vi "Registry.vi"(6 "Registry Configuration":T2, 7 "Command (Get)":T4, 8 "Use Regex? (F)":bool, 9 "UniqueName Object (Set)":refnum<class "UniqueName.lvclass">, 10 "Search term (Get & Delete Operations)":string, 11 "Key (FQN)":T3) -> (0 "Found or Completed?":bool, 1 "Returned Object":refnum<class "UniqueName.lvclass">, 2 "Multiple Match?":bool, 3 "Returned Objects":refnum<class "UniqueName.lvclass">[](array[class]), 4 "Registry Status":T1)   [LabVIEW 2014, in "UniqueName.lvlib" / "UniqueName.lvclass"]
uses:
  UniqueName.lvclass
  Command.ctl
  Key.ctl
  RegistryConfiguration.ctl
  Delimiter/Delimiter.lvclass
  RandomStringGenerator/RandomStringGenerator.lvclass
  UniquenessCriteria/UniquenessCriteria.lvclass
  NameIncrementAlgorithm/StringIncrementAlgorithm.lvclass
  RegistryStatus.ctl
  UniqueName.lvclass/UniqueName.ctl
  <vilib>/regexp/Match Regular Expression.xnode
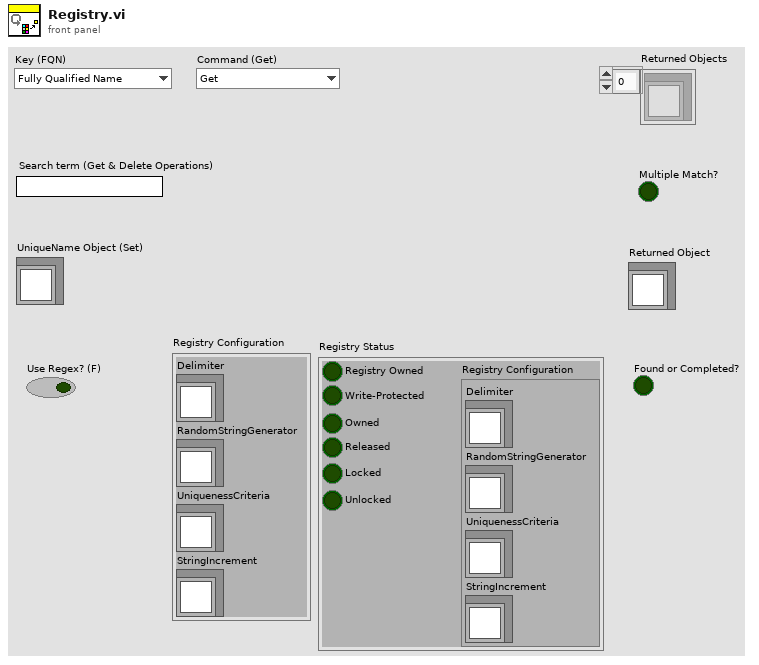
[diagram p1: front panel]
types:
  T1 = typedef "UniqueName.lvlib/UniqueName.lvclass/RegistryStatus.ctl" = cluster{"Registry Configuration":T2, "Registry Owned":bool, "Write-Protected":bool, "Owned":bool, "Released":bool, "Locked":bool, "Unlocked":bool}
  T2 = typedef "UniqueName.lvlib/UniqueName.lvclass/RegistryConfiguration.ctl" = cluster{"Delimiter":refnum<class "Delimiter.lvclass">, "RandomStringGenerator":refnum<class "RandomStringGenerator.lvclass">, "UniquenessCriteria":refnum<class "UniquenessCriteria.lvclass">, "StringIncrement":refnum<class "StringIncrementAlgorithm.lvclass">}
  T3 = typedef "UniqueName.lvlib/UniqueName.lvclass/Key.ctl" = enum16{"Fully Qualified Name", "Unique Name", "Given Name", "Parent Fully Qualified Name"}
  T4 = typedef "UniqueName.lvlib/UniqueName.lvclass/Command.ctl" = enum16{"Get", "Get All", "Set", "Delete", "Get Status", "Init", "Reserve Ownership", "Release Ownership", "Lock", "Unlock"}
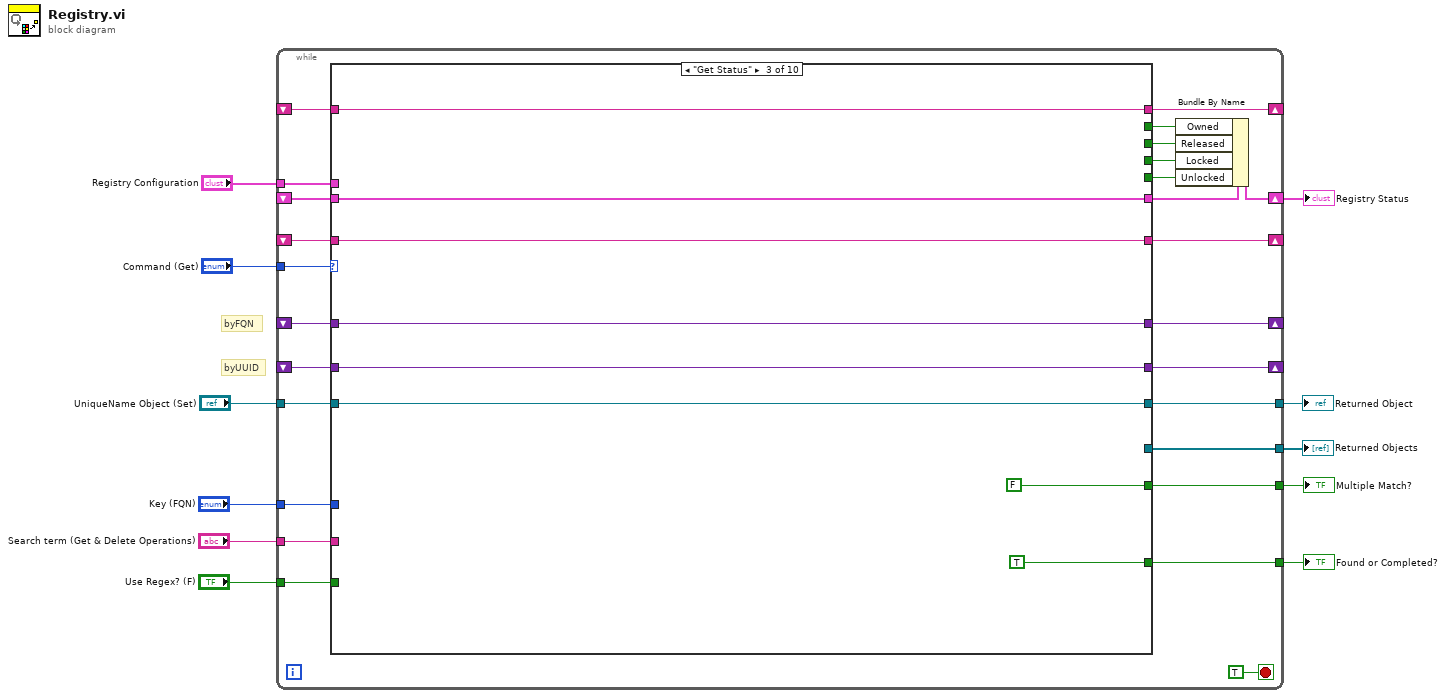
[diagram p0: block diagram]
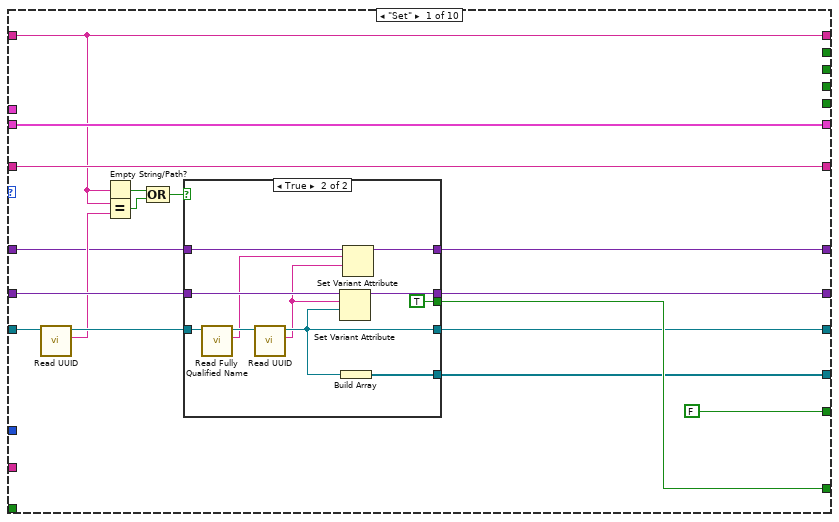
[diagram p2: hidden frame]
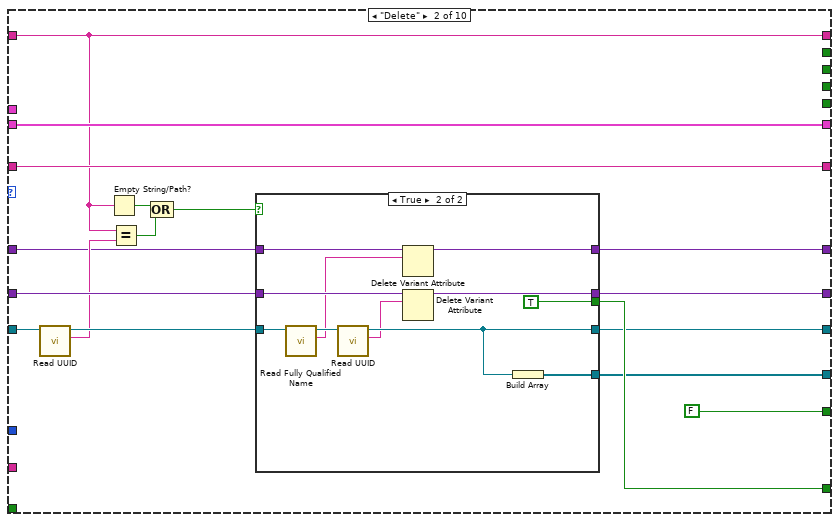
[diagram p4: hidden frame]
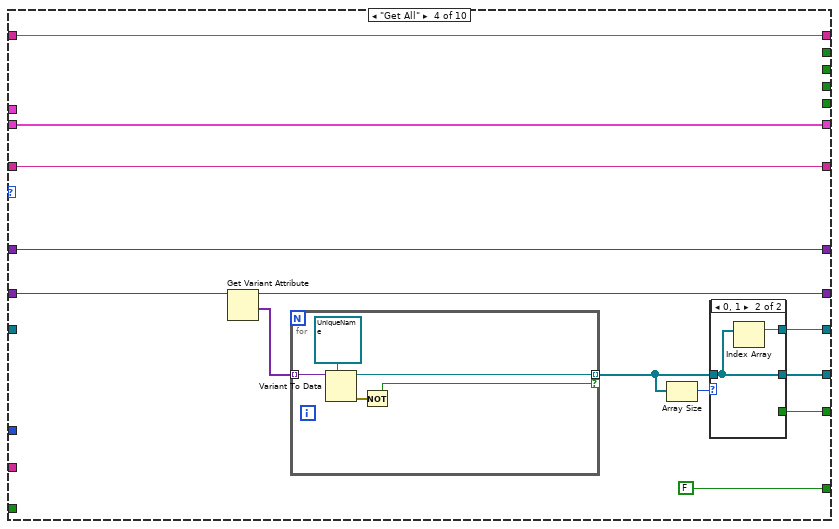
[diagram p6: hidden frame]
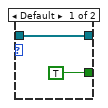
[diagram p7: hidden frame]
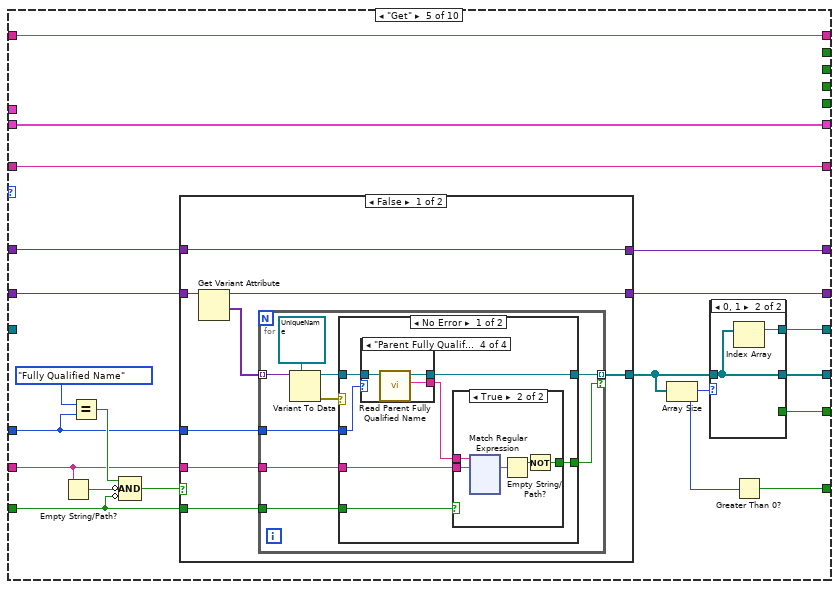
[diagram p8: hidden frame]
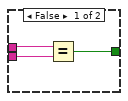
[diagram p9: hidden frame]
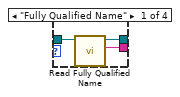
[diagram p10: hidden frame]
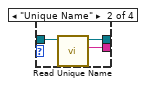
[diagram p11: hidden frame]
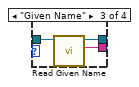
[diagram p12: hidden frame]
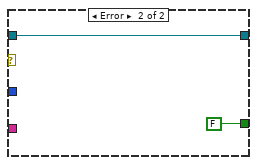
[diagram p13: hidden frame]
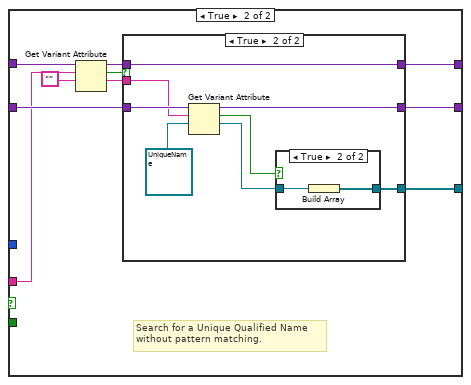
[diagram p14: hidden frame]
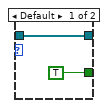
[diagram p17: hidden frame]
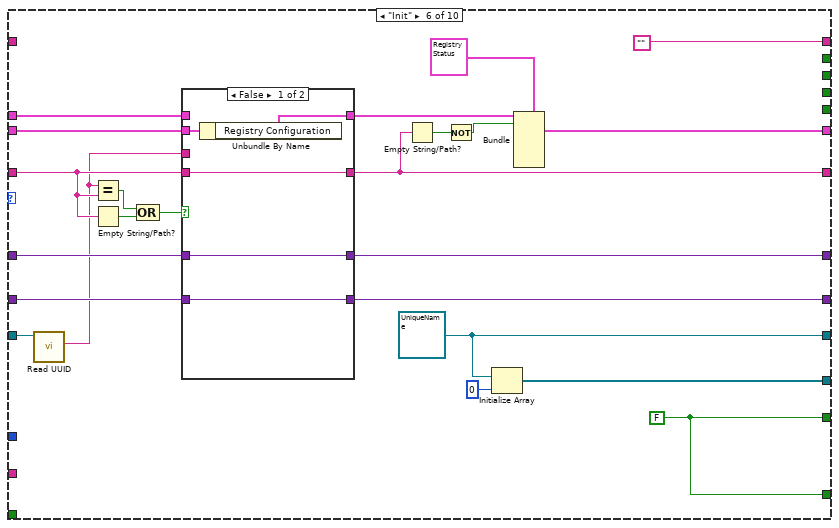
[diagram p18: hidden frame]
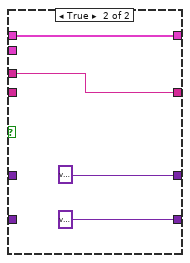
[diagram p19: hidden frame]
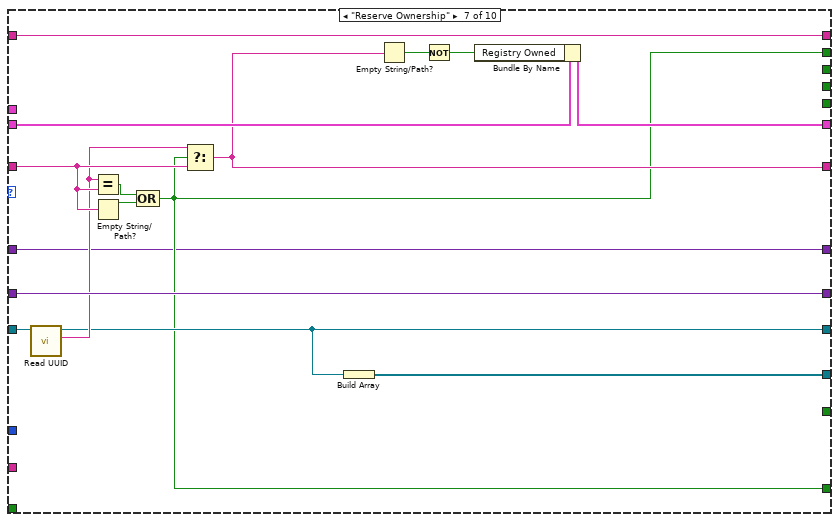
[diagram p20: hidden frame]
diagram:
  # "byUUID"
  # "byFQN"
  n1 = while {
    shift-right: [w35] -> _
    shift-left: _ -> [w33]
    tunnel: "Command (Get)" -> [w36]
    tunnel: "UniqueName Object (Set)" -> [w34]
    tunnel: [w32] -> w10
    tunnel: [w31] -> w9
    tunnel: [w30] -> w8
    tunnel: "Key (FQN)" -> [w29]
    tunnel: "Search term (Get & Delete Operations)" -> [w28]
    tunnel: [w27] -> w5
    tunnel: "Use Regex? (F)" -> [w26]
    shift-right: [w24] -> _
    shift-left: _ -> [w25]
    shift-right: [w19] -> w2
    shift-left: _ -> [w23]
    tunnel: "Registry Configuration" -> [w22]
    shift-right: [w20] -> _
    shift-left: _ -> [w21]
    shift-right: [w12] -> _
    shift-left: _ -> [w13]
    stop <- TRUE stop-if-true
    n2 = case shown="\"Get Status\"" w36 {
      tunnel: [w53 w83 w104 w116 w146 w356 w379 w396 w413 w429] -> w35
      tunnel: w34 -> [w46 w72 w105 _ _ w335 w371 w386 w401 w420]
      tunnel: w33 -> [w54 w84 w104 w117 w147 w348 w379 w396 w413 w429]
      tunnel: [w49 w80 w105 w110 w142 w355 w369 w385 w400 w415] -> w32
      tunnel: [w50 w77 _ w112 w144 w353 w368 _ _ w416] -> w31
      tunnel: [FALSE FALSE FALSE w111 w143 w352 _ _ _ FALSE] -> w30
      tunnel: w29 -> [_ _ _ _ w137 _ _ _ _ _]
      tunnel: w28 -> [_ _ _ _ w138 _ _ _ _ _]
      tunnel: [w52 w81 TRUE ("found") FALSE ("found") w134 w352 w367 w383 w398 w418] -> w27
      tunnel: w26 -> [_ _ _ _ w136 _ _ _ _ _]
      tunnel: w25 -> [w48 w79 w103 w109 w133 w347 w378 w395 w403 w428]
      tunnel: [w48 w79 w103 w109 w133 w341 w374 w395 w403 w423] -> w24
      tunnel: w23 -> [w47 w78 w102 w108 w132 w346 w376 w388 w405 w422]
      tunnel: [w47 w78 w102 w108 w132 w344 w375 w387 w404 w421] -> w18
      tunnel: w22 -> [_ _ _ _ _ w345 _ _ _ _]
      tunnel: w21 -> [w41 w75 w100 w107 w130 _ w377 w392 w410 w424]
      tunnel: [w41 w75 w100 w107 w130 "" w377 w389 w406 w424] -> w20
      tunnel: [_ _ _ _ _ _ _ w383 _ _] -> w17
      tunnel: [_ _ _ _ _ _ _ _ w398 _] -> w16
      tunnel: [_ _ _ _ _ _ w367 _ _ _] -> w15
      tunnel: [_ _ _ _ _ _ _ _ _ w418] -> w14
      tunnel: w13 -> [w39 w69 w99 w106 w129 w336 w366 w382 w397 w414]
      tunnel: [w38 w68 w99 w106 w128 w337 w366 w382 w397 w414] -> w12
      frame "Set" {
        n3 = call "Read UUID.vi"("UniqueName in"=w46) -> ("UUID"=w40:string, "UniqueName out"=w45:refnum<class "UniqueName.lvclass">)  [unwired: 9 in]
        n4 = Empty String/Path?(string/path=w41) -> (empty?=w42:bool)
        n5 = Equal?(x=w41, y=w40) -> (x = y?=w44:bool)
        n6 = Compound Arithmetic op=OR(w42, w44) -> (w43:bool)
        n7 = case shown="True" w43 {
          tunnel: w54 -> [w56 w67]
          tunnel: [w56 w66] -> w53
          tunnel: [_ TRUE ("replaced")] -> w52
          tunnel: w45 -> [_ w62]
          tunnel: [_ w65] -> w50
          tunnel: [_ w60] -> w49
          tunnel: w39 -> [w55 w63]
          tunnel: [w55 w57] -> w38
          frame False {
          }
          frame True {
            n8 = call "Read Fully Qualified Name.vi"("UniqueName in"=w62) -> ("Fully Qualified Name"=w59:string, "UniqueName out"=w61:refnum<class "UniqueName.lvclass">)  [unwired: 9 in]
            n9 = call "Read UUID.vi"("UniqueName in"=w61) -> ("UUID"=w58:string, "UniqueName out"=w60:refnum<class "UniqueName.lvclass">)  [unwired: 9 in]
            n10 = Set Variant Attribute(Variant=w67, name=w58, value=w60) -> (Variant out=w66:variant)  [unwired: 1 in, 2 out]
            n11 = Build Array(w60) -> (w65:refnum<class "UniqueName.lvclass">[])
            n12 = Set Variant Attribute(Variant=w63, name=w59, value=w58) -> (Variant out=w57:variant)  [unwired: 1 in, 2 out]
          }
        }
      }
      frame "Delete" {
        n13 = call "Read UUID.vi"("UniqueName in"=w72) -> ("UUID"=w70:string, "UniqueName out"=w71:refnum<class "UniqueName.lvclass">)  [unwired: 9 in]
        n14 = Empty String/Path?(string/path=w75) -> (empty?=w76:bool)
        n15 = Equal?(x=w75, y=w70) -> (x = y?=w74:bool)
        n16 = Compound Arithmetic op=OR(w76, w74) -> (w73:bool)
        n17 = case shown="True" w73 {
          tunnel: w71 -> [_ w90]
          tunnel: w84 -> [w86 w97]
          tunnel: [w86 w96] -> w83
          tunnel: [_ TRUE] -> w81
          tunnel: [_ w89] -> w80
          tunnel: [_ w94] -> w77
          tunnel: w69 -> [w85 w93]
          tunnel: [w85 w92] -> w68
          frame False {
          }
          frame True {
            n18 = call "Read Fully Qualified Name.vi"("UniqueName in"=w90) -> ("Fully Qualified Name"=w88:string, "UniqueName out"=w91:refnum<class "UniqueName.lvclass">)  [unwired: 9 in]
            n19 = call "Read UUID.vi"("UniqueName in"=w91) -> ("UUID"=w87:string, "UniqueName out"=w89:refnum<class "UniqueName.lvclass">)  [unwired: 9 in]
            n20 = Delete Variant Attribute(6:w88, 7:w93) -> (3:w92:variant)  [unwired: 1 in, 2 out]
            n21 = Delete Variant Attribute(6:w87, 7:w97) -> (3:w96:variant)  [unwired: 1 in, 2 out]
            n22 = Build Array(w89) -> (w94:refnum<class "UniqueName.lvclass">[])
          }
        }
      }
      frame "Get Status" {
      }
      frame "Get All" {
        n23 = Get Variant Attribute(Variant=w117) -> (duplicate Variant=w116:variant, values=w115:variant[])  [unwired: 3 in, 2 out]
        n24 = for {
          tunnel: w115 -> [w127] mode=indexing
          tunnel: [w125] -> w113 mode=indexing if=w123
          n25 = Variant To Data(type=refnum<class "UniqueName.lvclass"> refnum ("UniqueName.lvclass"), Variant=w127) -> (data=w125:refnum<class "UniqueName.lvclass">, error out=w124:errorcluster)  [unwired: 1 in]
          n26 = Not(x=w124) -> (.not. x?=w123:bool)
        }
        n27 = Array Size(array=w113) -> (size(s)=w114:i32)
        n28 = case shown="0, 1" w114 {
          tunnel: w113 -> [w120 w122]
          tunnel: [w120 w122] -> w112
          tunnel: [TRUE _] -> w111
          tunnel: [_ w121] -> w110
          frame Default {
          }
          frame 0, 1 {
            n29 = Index Array(array=w122) -> (element=w121:refnum<class "UniqueName.lvclass">)  [unwired: 1 in]
          }
        }
      }
      frame "Get" {
        n30 = Empty String/Path?(string/path=w138) -> (empty?=w141:bool)
        n31 = Equal?(x=Key."Fully Qualified Name", y=w137) -> (x = y?=w140:bool)
        n32 = Compound Arithmetic op=AND(w140, invert w141, invert w136) -> (w139:bool)
        n33 = case shown="False" w139 {
          tunnel: w147 -> [w155 w317]
          tunnel: [w154 w316] -> w146
          tunnel: [w153 w315] -> w145
          tunnel: w138 -> [w150 w312]
          tunnel: w137 -> [w149 _]
          tunnel: w136 -> [w151 _]
          tunnel: w129 -> [w148 w314]
          tunnel: [w148 w309] -> w128
          frame False {
            n34 = Get Variant Attribute(Variant=w155) -> (duplicate Variant=w154:variant, values=w152:variant[])  [unwired: 3 in, 2 out]
            n35 = for {
              tunnel: w152 -> [w164] mode=indexing
              tunnel: [w160] -> w153 mode=indexing if=w158
              tunnel: w151 -> [w157]
              tunnel: w150 -> [w156]
              tunnel: w149 -> [w162]
              n36 = Variant To Data(type=refnum<class "UniqueName.lvclass"> refnum ("UniqueName.lvclass"), Variant=w164) -> (data=w161:refnum<class "UniqueName.lvclass">, error out=w159:errorcluster)  [unwired: 1 in]
              n37 = case shown="No Error" w159 {
                tunnel: [w165 FALSE] -> w158
                tunnel: w162 -> [w171 _]
                tunnel: w161 -> [w170 w307]
                tunnel: [w169 w307] -> w160
                tunnel: w157 -> [w168 _]
                tunnel: w156 -> [w166 _]
                frame No Error {
                  n38 = case shown="\"Parent Fully Qualified Name\"" w171 {
                    tunnel: w170 -> [w296 w299 w302 w305]
                    tunnel: [w295 w298 w301 w304] -> w169
                    tunnel: [w294 w297 w300 w303] -> w167
                    frame "Fully Qualified Name" {
                      n39 = call "Read Fully Qualified Name.vi"("UniqueName in"=w296) -> ("Fully Qualified Name"=w294:string, "UniqueName out"=w295:refnum<class "UniqueName.lvclass">)  [unwired: 9 in]
                    }
                    frame "Unique Name" {
                      n40 = call "Read Unique Name.vi"("UniqueName in"=w299) -> ("Unique Name"=w297:string, "UniqueName out"=w298:refnum<class "UniqueName.lvclass">)  [unwired: 9 in]
                    }
                    frame "Given Name" {
                      n41 = call "Read Given Name.vi"("UniqueName in"=w302) -> ("Given Name"=w300:string, "UniqueName out"=w301:refnum<class "UniqueName.lvclass">)  [unwired: 9 in]
                    }
                    frame "Parent Fully Qualified Name" {
                      n42 = call "Read Parent Fully Qualified Name.vi"("UniqueName in"=w305) -> ("Parent Fully Qualified Name"=w303:string, "UniqueName out"=w304:refnum<class "UniqueName.lvclass">)  [unwired: 9 in]
                    }
                  }
                  n43 = case shown="True" w168 {
                    tunnel: w167 -> [w174 w179]
                    tunnel: w166 -> [w173 w178]
                    tunnel: [w172 w175] -> w165
                    frame False {
                      n44 = Equal?(x=w174, y=w173) -> (x = y?=w172:bool)
                    }
                    frame True {
                      n45 = xnode "Match Regular Expression"("input string"=w179, "regular expression"=w178) -> ("whole match"=w177:string)  [unwired: 4 in, 4 out]
                      n46 = Empty String/Path?(string/path=w177) -> (empty?=w176:bool)
                      n47 = Not(x=w176) -> (.not. x?=w175:bool)
                    }
                  }
                }
                frame Error {
                }
              }
            }
          }
          frame True {
            # "Search for a Unique Qualified Name\nwithout pattern matching."
            n48 = Get Variant Attribute(Variant=w314, name=w312, default value (empty Variant)="") -> (duplicate Variant=w308:variant, found=w310:bool, value=w311:string)  [unwired: 1 in, 1 out]
            n49 = case shown="True" w310 {
              tunnel: w317 -> [w318 w327]
              tunnel: [w318 w326] -> w316
              tunnel: [_ w324] -> w315
              tunnel: w311 -> [_ w322]
              tunnel: [w319 w320] -> w309
              tunnel: w308 -> [w319 w320]
              frame False {
              }
              frame True {
                n50 = Get Variant Attribute(Variant=w327, name=w322, default value (empty Variant)=refnum<class "UniqueName.lvclass"> refnum ("UniqueName Object (Set)")) -> (duplicate Variant=w326:variant, found=w323:bool, value=w325:refnum<class "UniqueName.lvclass">)  [unwired: 1 in, 1 out]
                n51 = case shown="True" w323 {
                  tunnel: w325 -> [_ w329]
                  tunnel: [_ w328] -> w324
                  frame False {
                  }
                  frame True {
                    n52 = Build Array(w329) -> (w328:refnum<class "UniqueName.lvclass">[])
                  }
                }
              }
            }
          }
        }
        n53 = Array Size(array=w145) -> (size(s)=w135:i32)
        n54 = case shown="0, 1" w135 {
          tunnel: w145 -> [w331 w333]
          tunnel: [w331 w333] -> w144
          tunnel: [TRUE _] -> w143
          tunnel: [_ w332] -> w142
          frame Default {
          }
          frame 0, 1 {
            n55 = Index Array(array=w333) -> (element=w332:refnum<class "UniqueName.lvclass">)  [unwired: 1 in]
          }
        }
        n56 = Greater Than 0?(x=w135) -> (x > 0?=w134:bool)
      }
      frame "Init" {
        w352 = FALSE
        w355 = refnum<class "UniqueName.lvclass"> refnum ("UniqueName Object (Set)")
        n57 = call "Read UUID.vi"("UniqueName in"=w335) -> ("UUID"=w334:string)  [unwired: 9 in, 1 out]
        n58 = Equal?(x=w334, y=w347) -> (x = y?=w350:bool)
        n59 = Empty String/Path?(string/path=w347) -> (empty?=w351:bool)
        n60 = Compound Arithmetic op=OR(w350, w351) -> (w349:bool)
        n61 = case shown="False" w349 {
          tunnel: [w361 variant] -> w356
          tunnel: w348 -> [w361 _]
          tunnel: [w360 w364] -> w341
          tunnel: w347 -> [w360 _]
          tunnel: w334 -> [_ w364]
          tunnel: w346 -> [w359 _]
          tunnel: w345 -> [_ w363]
          tunnel: [w358 w363] -> w339
          tunnel: [w357 variant] -> w337
          tunnel: w336 -> [w357 _]
          frame False {
            n62 = Unbundle By Name(w359) -> ("Registry Configuration"=w358:T2)
          }
          frame True {
          }
        }
        n63 = Empty String/Path?(string/path=w341) -> (empty?=w342:bool)
        n64 = Not(x=w342) -> (.not. x?=w338:bool)
        n65 = Initialize Array(w355, 0 ("dimension size")) -> (w353:refnum<class "UniqueName.lvclass">[])
        n66 = Bundle(cluster=T1 {"Registry Configuration"={"Delimiter"=refnum, "RandomStringGenerator"=refnum, "UniquenessCriteria"=refnum, "StringIncrement"=refnum}, "Registry Owned"=FALSE, "Write-Protected"=FALSE, "Owned"=FALSE, "Released"=FALSE, "Locked"=FALSE, "Unlocked"=FALSE} ("Status"), "Registry Configuration"=w339, "Registry Owned"=w338) -> (w344:T1)  [unwired: 5 in]
      }
      frame "Reserve Ownership" {
        n67 = call "Read UUID.vi"("UniqueName in"=w371) -> ("UUID"=w370:string, "UniqueName out"=w369:refnum<class "UniqueName.lvclass">)  [unwired: 9 in]
        n68 = Equal?(x=w370, y=w378) -> (x = y?=w380:bool)
        n69 = Empty String/Path?(string/path=w378) -> (empty?=w381:bool)
        n70 = Compound Arithmetic op=OR(w380, w381) -> (w367:bool)
        n71 = Select(t=w370, s=w367, f=w378) -> (s? t:f=w374:string)
        n72 = Build Array(w369) -> (w368:refnum<class "UniqueName.lvclass">[])
        n73 = Empty String/Path?(string/path=w374) -> (empty?=w373:bool)
        n74 = Not(x=w373) -> (.not. x?=w372:bool)
        n75 = Bundle By Name(cluster=w376, "Registry Owned"=w372) -> (w375:T1)
      }
      frame "Lock" {
        n76 = call "Read UUID.vi"("UniqueName in"=w386) -> ("UUID"=w384:string, "UniqueName out"=w385:refnum<class "UniqueName.lvclass">)  [unwired: 9 in]
        n77 = Equal?(x=w384, y=w392) -> (x = y?=w393:bool)
        n78 = Empty String/Path?(string/path=w392) -> (empty?=w394:bool)
        n79 = Compound Arithmetic op=OR(w393, w394) -> (w383:bool)
        n80 = Select(t=w384, s=w383, f=w392) -> (s? t:f=w389:string)
        n81 = Empty String/Path?(string/path=w389) -> (empty?=w391:bool)
        n82 = Not(x=w391) -> (.not. x?=w390:bool)
        n83 = Bundle By Name(cluster=w388, "Write-Protected"=w390) -> (w387:T1)
      }
      frame "Unlock" {
        # "Owner can unlock"
        n84 = call "Read UUID.vi"("UniqueName in"=w401) -> ("UUID"=w399:string, "UniqueName out"=w400:refnum<class "UniqueName.lvclass">)  [unwired: 9 in]
        n85 = Equal?(x=w399, y=w403) -> (x = y?=w402:bool)
        n86 = Equal?(x=w399, y=w410) -> (x = y?=w411:bool)
        n87 = Empty String/Path?(string/path=w410) -> (empty?=w412:bool)
        n88 = Compound Arithmetic op=OR(w411, w412, w402) -> (w398:bool)
        n89 = Select(t="", s=w398, f=w410) -> (s? t:f=w406:string)
        n90 = Empty String/Path?(string/path=w406) -> (empty?=w408:bool)
        n91 = Not(x=w408) -> (.not. x?=w407:bool)
        n92 = Bundle By Name(cluster=w405, "Write-Protected"=w407) -> (w404:T1)
      }
      frame "Release Ownership" {
        n93 = call "Read UUID.vi"("UniqueName in"=w420) -> ("UUID"=w419:string, "UniqueName out"=w415:refnum<class "UniqueName.lvclass">)  [unwired: 9 in]
        n94 = Equal?(x=w419, y=w428) -> (x = y?=w430:bool)
        n95 = Empty String/Path?(string/path=w428) -> (empty?=w431:bool)
        n96 = Compound Arithmetic op=OR(w430, w431) -> (w418:bool)
        n97 = Select(t="", s=w418, f=w428) -> (s? t:f=w423:string)
        n98 = Empty String/Path?(string/path=w423) -> (empty?=w426:bool)
        n99 = Not(x=w426) -> (.not. x?=w425:bool)
        n100 = Bundle By Name(cluster=w422, "Registry Owned"=w425) -> (w421:T1)
        n101 = Build Array(w415) -> (w416:refnum<class "UniqueName.lvclass">[])
      }
    }
    n102 = Bundle By Name(cluster=w18, "Owned"=w15, "Released"=w14, "Locked"=w17, "Unlocked"=w16) -> (w19:T1)
  }
  "Returned Object" <- w10
  "Returned Objects" <- w9
  "Multiple Match?" <- w8
  "Found or Completed?" <- w5
  "Registry Status" <- w2
